vi "Module_KEITHLEY2470.vi"(7 "cmd":T2, 8 "error in (no error)":errorcluster, 11 "Cluster":T1={"VISA resource name"="", "Function (0: Volts) 1"=1, "Function (0: Volts) 2 "=0, "Enable Auto Range (T:Enable)"=TRUE, "Source Mode  (0: Voltage)"=0, "Source Level (0)"=0.0, "Source Limit Level (0.1)"=0.01} {"Source Limit Level (0.1)" format="%#_13g"; "Source Level (0)" format="%#_13g"; "Source Mode  (0: Voltage)" items=["Voltage", "Current"]; "Function (0: Volts) 2" items=["Volts", "Current", "Resistance"]; "Function (0: Volts) 1" items=["Volts", "Current", "Resistance"]}) -> (0 "error out":errorcluster, 3 "data":dbl[](array[numeric]))   [LabVIEW 2019]
uses:
  Type Definition/cnt_keithley.ctl
  Type Definition/handle_Para.ctl
  <instrlib>/Keithley 2450/Keithley 2450.lvlib
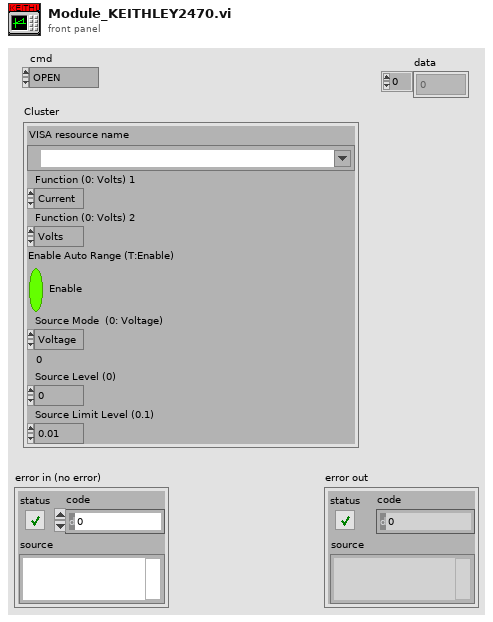
[diagram p1: front panel]
types:
  T1 = typedef "handle_Para.ctl" = cluster{"VISA resource name":refnum<visa-resource-name>, "Function (0: Volts) 1":u16, "Function (0: Volts) 2 ":u16, "Enable Auto Range (T:Enable)":bool, "Source Mode  (0: Voltage)":u16, "Source Level (0)":dbl, "Source Limit Level (0.1)":dbl}
  T2 = typedef "cnt_keithley.ctl" = enum16{"OPEN", "SET", "LEVEL", "ON", "OFF", "CLOSE", "READ", "DEFUALT"}
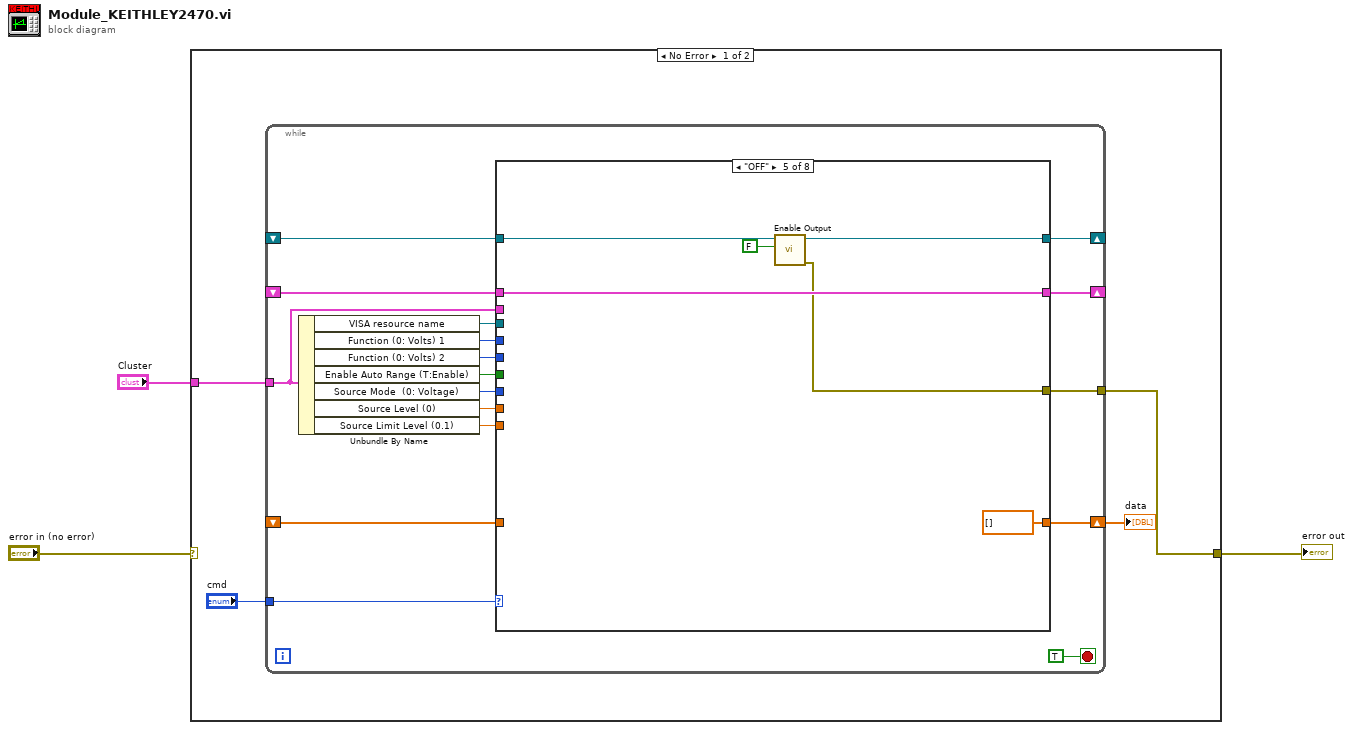
[diagram p0: block diagram]
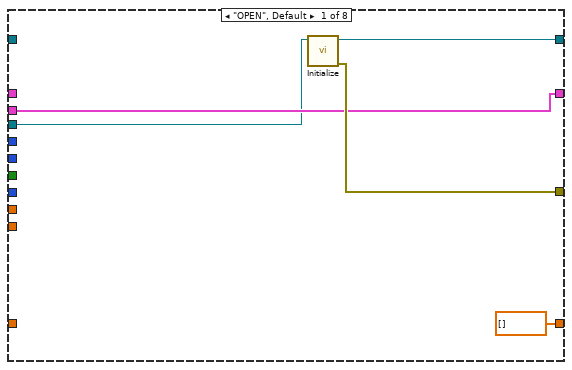
[diagram p2: hidden frame]
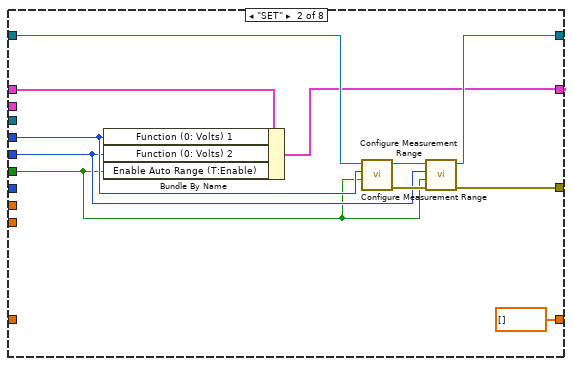
[diagram p3: hidden frame]
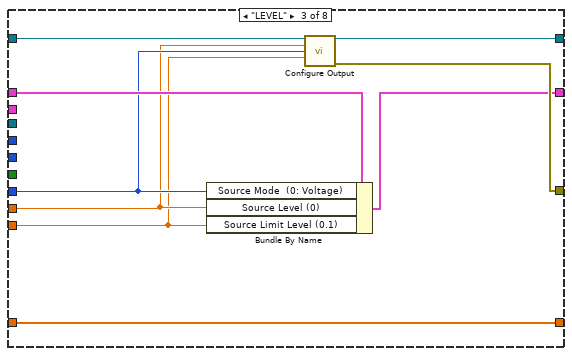
[diagram p4: hidden frame]
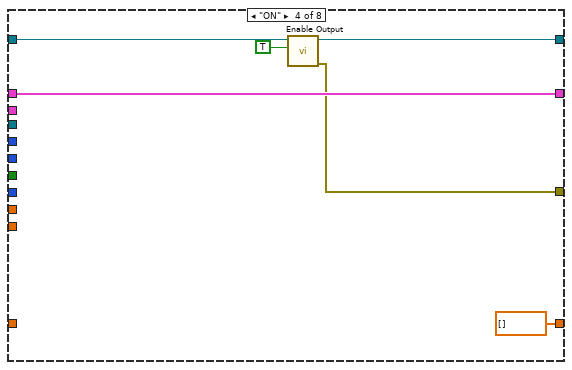
[diagram p5: hidden frame]
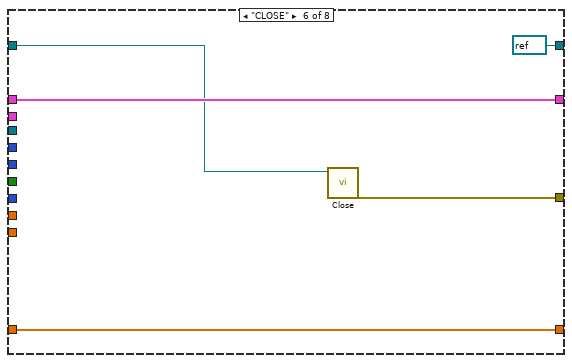
[diagram p6: hidden frame]
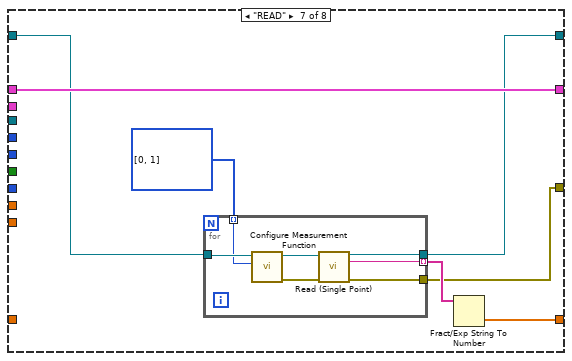
[diagram p7: hidden frame]
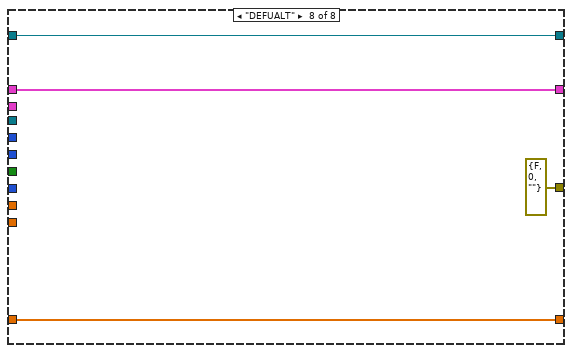
[diagram p8: hidden frame]
diagram:
  n1 = case shown="No Error" "error in (no error)" {
    selector: "error in (no error)" -> [_ w85]
    tunnel: [w6 w85] -> w2
    tunnel: "Cluster" -> [w5 _]
    frame No Error {
      n2 = while {
        tunnel: "cmd" -> [w23]
        shift-right: [w22] -> _
        shift-left: _ -> [w21]
        tunnel: [w20] -> w6
        shift-right: [w19] -> _
        shift-left: _ -> [w18]
        tunnel: w5 -> [w9]
        shift-right: [w11] -> w4
        shift-left: _ -> [w10]
        stop <- TRUE stop-if-true
        n3 = Unbundle By Name(w9) -> ("VISA resource name"=w8:refnum<visa-resource-name>, "Function (0: Volts) 1"=w17:u16, "Function (0: Volts) 2"=w16:u16, "Enable Auto Range (T:Enable)"=w15:bool, "Source Mode  (0: Voltage)"=w14:u16, "Source Level (0)"=w13:dbl, "Source Limit Level (0.1)"=w12:dbl)
        n4 = case shown="\"OFF\"" w23 {
          tunnel: [w29 w37 w48 w52 w58 refnum<visa-resource-name> refnum ("VISA resource name out") w69 w84] -> w22
          tunnel: w21 -> [_ w38 w49 w53 w59 w65 w70 w84]
          tunnel: [w28 w36 w47 w51 w57 w64 w68 errorcluster {"status"=FALSE, "code"=0, "source"=""} ("error out")] -> w20
          tunnel: [w26 w34 w42 w55 w61 w66 w73 w83] -> w19
          tunnel: w18 -> [_ w35 w46 w55 w61 w66 w73 w83]
          tunnel: w17 -> [_ w33 _ _ _ _ _ _]
          tunnel: w16 -> [_ w32 _ _ _ _ _ _]
          tunnel: w15 -> [_ w31 _ _ _ _ _ _]
          tunnel: w14 -> [_ _ w45 _ _ _ _ _]
          tunnel: w13 -> [_ _ w44 _ _ _ _ _]
          tunnel: w12 -> [_ _ w43 _ _ _ _ _]
          tunnel: [dbl[] [] dbl[] [] w41 dbl[] [] dbl[] [] w62 w67 w82] -> w11
          tunnel: w10 -> [_ _ w41 _ _ w62 _ w82]
          tunnel: w9 -> [w26 _ _ _ _ _ _ _]
          tunnel: w8 -> [w25 _ _ _ _ _ _ _]
          frame "OPEN", Default {
            n5 = call <instrlib>:"Initialize.vi"("VISA resource name"=w25) -> ("error out"=w28:errorcluster, "VISA resource name out"=w29:refnum<visa-resource-name>)  [unwired: 9 in]
          }
          frame "SET" {
            n6 = Bundle By Name(cluster=w35, "Function (0: Volts) 1"=w33, "Function (0: Volts) 2"=w32, "Enable Auto Range (T:Enable)"=w31) -> (w34:T1)
            n7 = call <instrlib>:"Configure Measurement Range.vi"("Enable Auto Range (T:Enable)"=w31, "Function (0: Volts)"=w33, "VISA resource name"=w38) -> ("error out"=w39:errorcluster, "VISA resource name out"=w40:refnum<visa-resource-name>)  [unwired: 7 in]
            n8 = call <instrlib>:"Configure Measurement Range.vi"("error in (no error)"=w39, "Enable Auto Range (T:Enable)"=w31, "Function (0: Volts)"=w32, "VISA resource name"=w40) -> ("error out"=w36:errorcluster, "VISA resource name out"=w37:refnum<visa-resource-name>)  [unwired: 6 in]
          }
          frame "LEVEL" {
            n9 = Bundle By Name(cluster=w46, "Source Mode  (0: Voltage)"=w45, "Source Level (0)"=w44, "Source Limit Level (0.1)"=w43) -> (w42:T1)
            n10 = call <instrlib>:"Configure Output.vi"("VISA resource name"=w49, "Source Level (0)"=w44, "Source Mode  (0: Voltage)"=w45, "Source Limit Level (0.1)"=w43) -> ("VISA resource name out"=w48:refnum<visa-resource-name>, "error out"=w47:errorcluster)  [unwired: 10 in]
          }
          frame "ON" {
            n11 = call <instrlib>:"Enable Output.vi"("Enable Output (T: Enable)"=TRUE, "VISA resource name"=w53) -> ("error out"=w51:errorcluster, "VISA resource name out"=w52:refnum<visa-resource-name>)  [unwired: 8 in]
          }
          frame "OFF" {
            n12 = call <instrlib>:"Enable Output.vi"("Enable Output (T: Enable)"=FALSE, "VISA resource name"=w59) -> ("error out"=w57:errorcluster, "VISA resource name out"=w58:refnum<visa-resource-name>)  [unwired: 8 in]
          }
          frame "CLOSE" {
            n13 = call <instrlib>:"Close.vi"("VISA resource name"=w65) -> ("error out"=w64:errorcluster)  [unwired: 10 in]
          }
          frame "READ" {
            w71 = u16[] [0, 1] items=["Volts", "Current", "Auto Resistance"]
            n14 = for {
              tunnel: w70 -> [w80]
              tunnel: [w79] -> w72 mode=indexing
              tunnel: [w78] -> w69
              tunnel: [w77] -> w68
              tunnel: w71 -> [w76] mode=indexing
              n15 = call <instrlib>:"Configure Measurement Function.vi"("Function (0: Volts)"=w76, "VISA resource name"=w80) -> ("error out"=w74:errorcluster, "VISA resource name out"=w75:refnum<visa-resource-name>)  [unwired: 8 in]
              n16 = call <instrlib>:"Read (Single Point).vi"("VISA resource name"=w75, "error in (no error)"=w74) -> ("VISA resource name out"=w78:refnum<visa-resource-name>, "Data out"=w79:string, "error out"=w77:errorcluster)  [unwired: 11 in]
            }
            n17 = Fract/Exp String To Number(string=w72) -> (number=w67:dbl[])  [unwired: 3 in, 1 out]
          }
          frame "DEFUALT" {
          }
        }
      }
      "data" <- w4
    }
    frame Error {
    }
  }
  "error out" <- w2
